vi "Init TS Results File.vi"(8 "error in":errorcluster, 11 "Generic Test Stand in":refnum<class "Generic Test Stand.lvclass">) -> (0 "error out":errorcluster, 3 "Generic Test Stand out":refnum<class "Generic Test Stand.lvclass">)   [LabVIEW 2019, in "Generic Test Stand.lvclass"]
uses:
  Generic Test Stand.lvclass
  Generic Test Stand.lvclass/Generic Test Stand.ctl
  DAC/DAC.lvclass
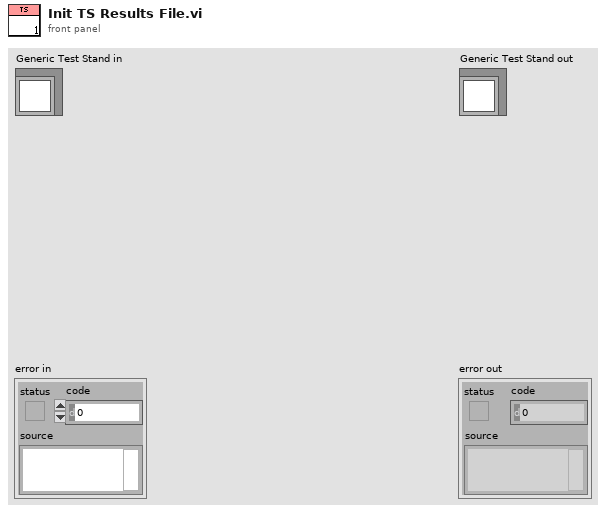
[diagram p1: front panel]
types:
  T1 = enum16{"open", "open or create", "create or replace", "create", "open (read-only)"}
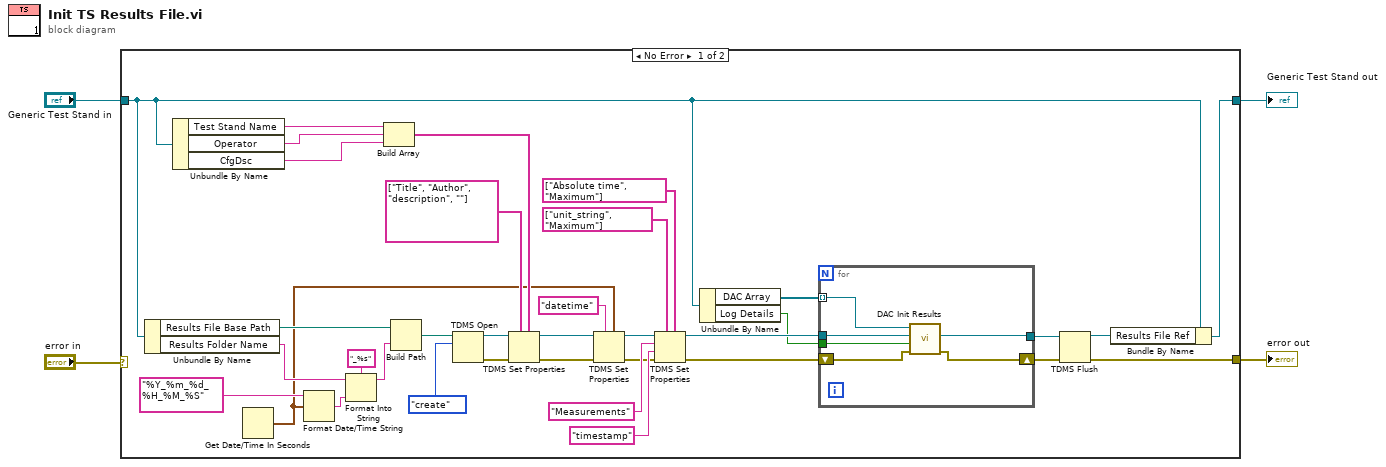
[diagram p0: block diagram]
diagram:
  n1 = case shown="No Error" "error in" {
    selector: "error in" -> [_ w47]
    tunnel: [w35 w47] -> w1
    tunnel: [w38 w46] -> w2
    tunnel: "Generic Test Stand in" -> [w29 w46]
    frame No Error {
      n2 = Unbundle By Name(w29) -> ("Results File Base Path"=w34:path, "Results Folder Name"=w14:string)
      n3 = Unbundle By Name(w29) -> ("Test Stand Name"=w28:string, "Operator"=w27:string, "CfgDsc"=w5:string)
      n4 = Get Date/Time In Seconds() -> (seconds since 1Jan1904=w6:timestamp)
      n5 = Format Date/Time String(time format string (%c)="%Y_%m_%d_%H_%M_%S", seconds (now)=w6) -> (date/time string=w12:string)  [unwired: 1 in]
      n6 = Format Into String(format string="_%s", initial string=w14, w12) -> (resulting string=w32:string)  [unwired: 1 in, 1 out]
      n7 = Build Array(w28, w27, w5) -> (w24:string[])
      n8 = Build Path(base path=w34, name or relative path=w32) -> (appended path=w31:path)
      n9 = TDMS Open(10:T1."create" ("operation (0:open)"), 11:w31) -> (0:w23:errorcluster, 3:w26:refnum<k34>)  [unwired: 5 in]
      n10 = TDMS Set Properties(5:w24, 7:string[] ["Title", "Author", "description", ""] ("property names"), 8:w23, 11:w26) -> (0:w10:errorcluster, 3:w11:refnum<k34>)  [unwired: 2 in, 2 out]
      n11 = TDMS Set Properties(5:w6, 7:"datetime", 8:w10, 11:w11) -> (0:w8:errorcluster, 3:w9:refnum<k34>)  [unwired: 2 in, 2 out]
      n12 = TDMS Set Properties(5:string[] ["Absolute time", "Maximum"] ("property names"), 7:string[] ["unit_string", "Maximum"] ("property names"), 8:w8, 9:"timestamp" ("channel name"), 10:"Measurements" ("group name in (Untitled)"), 11:w9) -> (0:w18:errorcluster, 3:w17:refnum<k34>)  [unwired: 2 out]
      n13 = Unbundle By Name(w29) -> ("DAC Array"=w39:refnum<class "DAC.lvclass">[], "Log Details"=w15:bool)
      n14 = for {
        tunnel: w39 -> [w41] mode=indexing
        shift-right: [w43] -> w36
        shift-left: w18 -> [w44]
        tunnel: w17 -> [w45]
        tunnel: [w42] -> w16
        tunnel: w15 -> [w40]
        n15 = call-dynamic "DAC Init Results.vi"("error in"=w44, "Log Details?"=w40, "tdms file"=w45, "DAC in"=w41) -> ("error out"=w43:errorcluster, "tdms file out"=w42:refnum<k34>)  [unwired: 6 in]
      }
      n16 = TDMS Flush(4:w36, 7:w16) -> (0:w35:errorcluster, 3:w37:refnum<k34>)
      n17 = Bundle By Name(cluster=w29, "Results File Ref"=w37) -> (w38:refnum<class "Generic Test Stand.lvclass">)
    }
    frame Error {
    }
  }
  "error out" <- w1
  "Generic Test Stand out" <- w2
